vi "Log Out.vi"(0 "session in":refnum<k21>, 5 "chassis":refnum<k21>, 11 "error in (no error)":errorcluster) -> (4 "session out":refnum<k21>, 15 "error out":errorcluster)   [LabVIEW 2020, in "SLSC.lvlib"]
doc: "Deletes any saved credentials for this chassis."
uses:
  <vilib>/SLSC/SLSC.lvlib
  nislsclvapi.dll
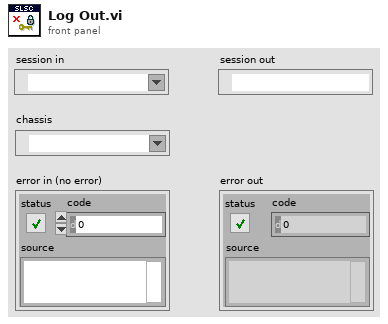
[diagram p1: front panel]
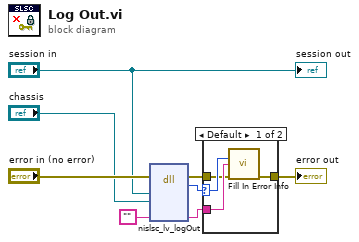
[diagram p0: block diagram]
diagram:
  n1 = dll-call lib="nislsclvapi.*" fn="nislsc_lv_logOut"(error in="error in (no error)", "session"="session in", "chassis"="chassis", "extendedErrorInfo"="") -> (error out=w5:errorcluster, "return type"=w4:i32, "extendedErrorInfo"=w3:string)  [unwired: 6 in, 1 out]
  n2 = case shown="Default" w4 {
    selector: w4 -> [w12 _]
    tunnel: w3 -> [w11 _]
    tunnel: w5 -> [w10 w13]
    tunnel: [w9 w13] -> w2
    frame Default {
      n3 = call <vilib>:"Fill In Error Info.vi"("status code"=w12, "extended error info"=w11, "error in"=w10) -> ("error out"=w9:errorcluster)  [unwired: 12 in]
    }
    frame 0 {
    }
  }
  "error out" <- w2
  "session out" <- "session in"
